vi "ComputeShift.vi"(0 "X1":dbl format="%#_11g", 1 "Y1":dbl format="%#_11g", 2 "X2":dbl format="%#_10g", 3 "Y2":dbl format="%#_11g", 4 "Dist Right":dbl, 6 "Dist Left":dbl) -> (7 "XShift":dbl format="%#_8g", 8 "YShift":dbl format="%#_8g", 9 "Length":dbl format="%#_9g")   [LabVIEW 2019]
panel:
  out "Ux":dbl
  out "Uy":dbl
  out "X_cp":dbl format="%#_8g"
  out "Y_cp":dbl format="%#_8g"
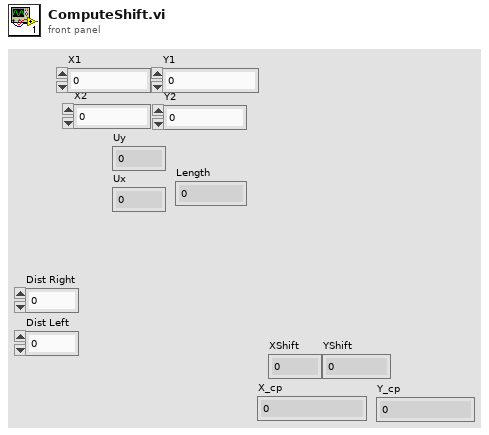
[diagram p1: front panel]
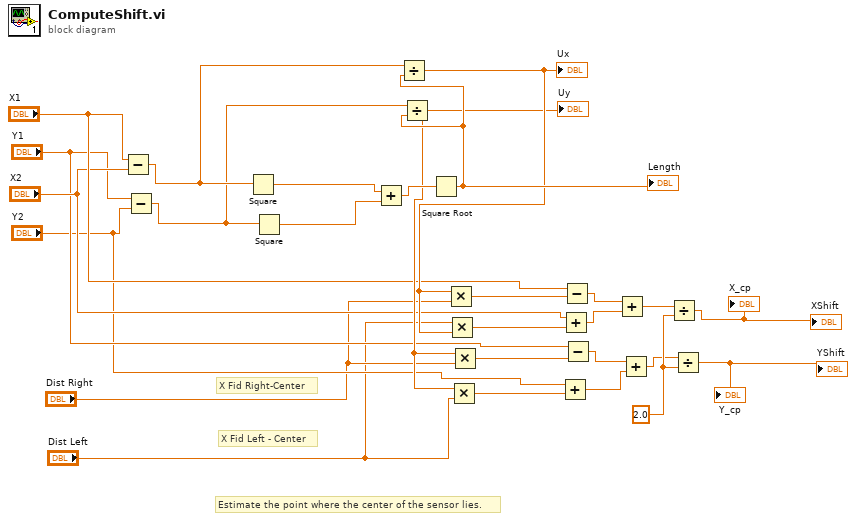
[diagram p0: block diagram]
diagram:
  w19 = 2.0 ("y")
  # "Estimate the point where the center of the sensor lies."
  # "X Fid Left - Center"
  # "X Fid Right-Center"
  n1 = Subtract(x="X1", y="X2") -> (x-y=w11:dbl)
  n2 = Subtract(x="Y1", y="Y2") -> (x-y=w10:dbl)
  n3 = Square(x=w11) -> (x^2=w13:dbl)
  n4 = Square(x=w10) -> (x^2=w12:dbl)
  n5 = Add(x=w13, y=w12) -> (x+y=w14:dbl)
  n6 = Square Root(x=w14) -> (sqrt(x)=w9:dbl)
  "Length" <- w9
  n7 = Divide(x=w11, y=w9) -> (x/y=w8:dbl)
  "Ux" <- w8
  n8 = Divide(x=w10, y=w9) -> (x/y=w7:dbl)
  "Uy" <- w7
  n9 = Multiply(x=w8, y="Dist Right") -> (x*y=w27:dbl)
  n10 = Multiply(x="Dist Left", y=w8) -> (x*y=w26:dbl)
  n11 = Multiply(x=w7, y="Dist Left") -> (x*y=w24:dbl)
  n12 = Multiply(x=w7, y="Dist Right") -> (x*y=w25:dbl)
  n13 = Add(x="Y2", y=w24) -> (x+y=w20:dbl)
  n14 = Add(x="X2", y=w26) -> (x+y=w22:dbl)
  n15 = Subtract(x="X1", y=w27) -> (x-y=w23:dbl)
  n16 = Subtract(x="Y1", y=w25) -> (x-y=w21:dbl)
  n17 = Add(x=w23, y=w22) -> (x+y=w17:dbl)
  n18 = Add(x=w21, y=w20) -> (x+y=w18:dbl)
  n19 = Divide(x=w17, y=w19) -> (x/y=→"XShift" →"X_cp":dbl)
  n20 = Divide(x=w18, y=w19) -> (x/y=→"YShift" →"Y_cp":dbl)
